vi "CreateBoard.vi"(8 "Error In":errorcluster, 9 "Param In":T1 caption="Main parameters", 10 "Arr Ref":refnum<vi>, 11 "Main VI Ref":refnum<vi>) -> (0 "Error Out":errorcluster, 1 "Param Out":T1 caption="Main parameters", 2 "Main Board":T2[][](array[typedef]))   [LabVIEW 2020]
doc: "Creates an main board and adjusts the dimensions and position of the main vi."
uses:
  Ctrls/ElementalCell.ctl
  Ctrls/MainData.ctl
  <vilib>/Utility/miscctls.llb/LVPositionTypeDef.ctl
  <vilib>/Utility/miscctls.llb/LVPointTypeDef.ctl
panel:
  in  "Boolean":T2
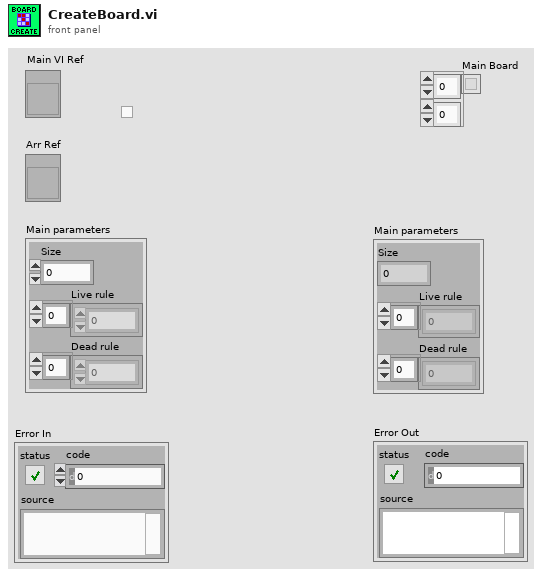
[diagram p1: front panel]
types:
  T1 = typedef "MainData.ctl" = cluster{"Size":i32, "Live rule":i32[], "Dead rule":i32[]}
  T2 = typedef "ElementalCell.ctl" = bool
  T3 = enum32{"Invalid", "Standard", "Closed", "Hidden", "Minimized", "Maximized"}
  T4 = typedef "LVPositionTypeDef.ctl" = cluster{"Left":i32, "Top":i32}
  T5 = typedef "LVBoundsTypeDef.ctl" = cluster{"Width":u32, "Height":u32}
  T6 = typedef "LVRectTypeDef.ctl" = cluster{"Left":i16, "Top":i16, "Right":i16, "Bottom":i16}
  T7 = typedef "LVPointTypeDef.ctl" = cluster{"Horizontal":i16, "Vertical":i16}
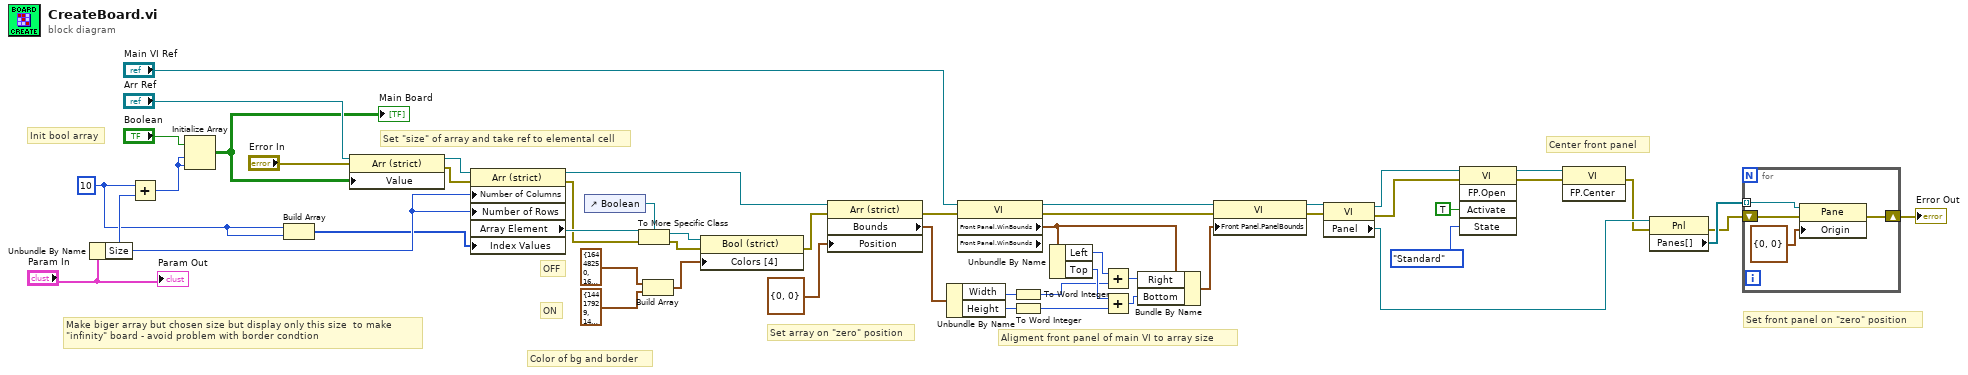
[diagram p0: block diagram]
diagram:
  w3 = 10 ("y")
  # "Make biger array but chosen size but display only this size  to make \n\"infinity\" board - avoid problem with border condtion"
  # "Center front panel"
  # "Set front panel on \"zero\" position"
  # "Set array on \"zero\" position"
  # "Aligment front panel of main VI to array size"
  # "Set \"size\" of array and take ref to elemental cell"
  # "ON"
  # "OFF"
  # "Color of bg and border"
  # "Init bool array"
  n1 = Unbundle By Name("Param In") -> ("Size"=w5:i32)
  n2 = Add(x=w3, y=w5) -> (x+y=w4:i32)
  n3 = Initialize Array("Boolean", w4, w4) -> (w23:T2[][])
  "Main Board" <- w23
  n4 = Build Array(w3, w3) -> (w2:i32[])
  n5 = property class="Arr (strict)"(reference="Arr Ref", error in="Error In", "Value"=w23) -> (reference out=w41:refnum<vi>, error out=w40:errorcluster)
  n6 = property on="Property Node" class="Arr (strict)"(reference=w41, error in=w40, "Number of Columns"=w5, "Number of Rows"=w5, "Index Values"=w2) -> (reference out=w22:refnum<vi>, error out=w46:errorcluster, "Array Element"=w49:refnum<vi>)
  n7 = control-ref of="Boolean"() -> (w47:refnum<vi>)
  n8 = To More Specific Class(target class=w47, reference=w49, error in=w46) -> (specific class reference=w50:refnum<vi>, error out=w45:errorcluster)
  n9 = Build Array(cluster{u32, u32} {16448250, 16448250}, cluster{u32, u32} {14417929, 14417929}) -> (w14:cluster{u32, u32}[])
  n10 = property class="Bool (strict)"(reference=w50, error in=w45, "Colors [4]"=w14) -> (error out=w39:errorcluster)  [unwired: 1 out]
  n11 = property class="Arr (strict)"(reference=w22, error in=w39, "Position"=T4 {"Left"=0, "Top"=0}) -> (error out=w29:errorcluster, "Bounds"=w28:T5)  [unwired: 1 out]
  n12 = Unbundle By Name(w28) -> ("Width"=w27:u32, "Height"=w26:u32)
  n13 = property class="VI" props=["Front Panel.WinBounds", "Front Panel.WinBounds"](reference="Main VI Ref", error in=w29) -> (reference out=w32:refnum<vi>, error out=w31:errorcluster, "Front Panel.WinBounds"=w33:T6)  [unwired: 1 out]
  n14 = To Word Integer(number=w27) -> (16bit integer=w36:i16)
  n15 = To Word Integer(number=w26) -> (16bit integer=w25:i16)
  n16 = Unbundle By Name(w33) -> ("Left"=w34:i16, "Top"=w37:i16)
  n17 = Add(x=w34, y=w36) -> (x+y=w35:i16)
  n18 = Add(x=w37, y=w25) -> (x+y=w24:i16)
  n19 = Bundle By Name(cluster=w33, "Right"=w35, "Bottom"=w24) -> (w38:T6)
  n20 = property class="VI"(reference=w32, error in=w31, "Front Panel.PanelBounds"=w38) -> (reference out=w21:refnum<vi>, error out=w12:errorcluster)
  n21 = property class="VI"(reference=w21, error in=w12) -> (reference out=w10:refnum<vi>, error out=w16:errorcluster, "Panel"=w17:refnum<vi>)
  n22 = invoke class="VI" method="FP.Open"(reference=w10, error in=w16, "Activate"=TRUE ("Activate?"), "State"=T3."Standard") -> (reference out=w9:refnum<vi>, error out=w11:errorcluster)  [unwired: 1 in, 3 out]
  n23 = invoke class="VI" method="FP.Center"(reference=w9, error in=w11) -> (error out=w15:errorcluster)  [unwired: 1 in, 2 out]
  n24 = property class="Pnl"(reference=w17, error in=w15) -> (error out=w19:errorcluster, "Panes[]"=w20:refnum<vi>[])  [unwired: 1 out]
  n25 = for {
    tunnel: w20 -> [w54] mode=indexing
    shift-right: [w51] -> w18
    shift-left: w19 -> [w53]
    n26 = property class="Pane"(reference=w54, error in=w53, "Origin"=T7 {"Horizontal"=0, "Vertical"=0}) -> (error out=w51:errorcluster)  [unwired: 1 out]
  }
  "Error Out" <- w18
  "Param Out" <- "Param In"
